vi "Comm@Write__Parameter.vi"(1 "ParamterIn":string) -> (0 "ParamterOut":string)   [LabVIEW 2019]
panel:
  in  "Message":string(combo)
  in  "Data2":string(combo) caption="Postfix"
  in  "Data1":string(combo) caption="Data"
  in  "CommName":string(combo)
  in  "Confirm":bool
  # "Comm@Write $Comm,$Data1,$Data2(,$[[label]]Message)"
  # "COM               $Data,$Postfix,$[[label]]Message)\nTCP                $Data,$Postfix,$[[label]]Message)\nServer              $Data,$Postfix,$[[label]]Message)\nModbus           $Address,$Data(,$[[label]]Message)\nModbus(TCP)   $Address,$Data(,$[[label]]Message)"
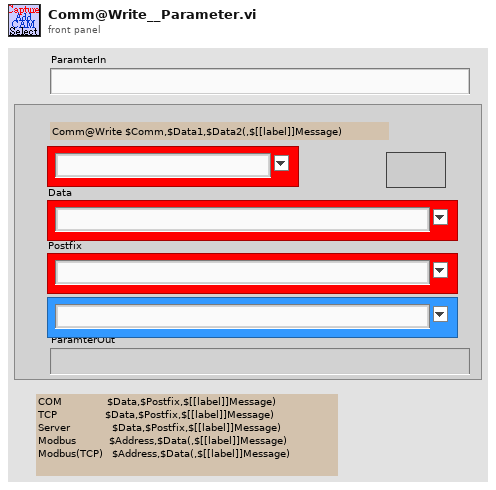
[diagram p1: front panel]
types:
  T1 = cluster{"Type":enum16{"COM", "TCP", "TCP(Slave)", "Modbus", "Modbus(TCP)", "COM(Slave)"}, "COMM":variant, "DataType":enum16{"ASCII", "Binary"}}
  T2 = enum16{"COM", "TCP", "TCP(Slave)", "Modbus", "Modbus(TCP)", "COM(Slave)"}
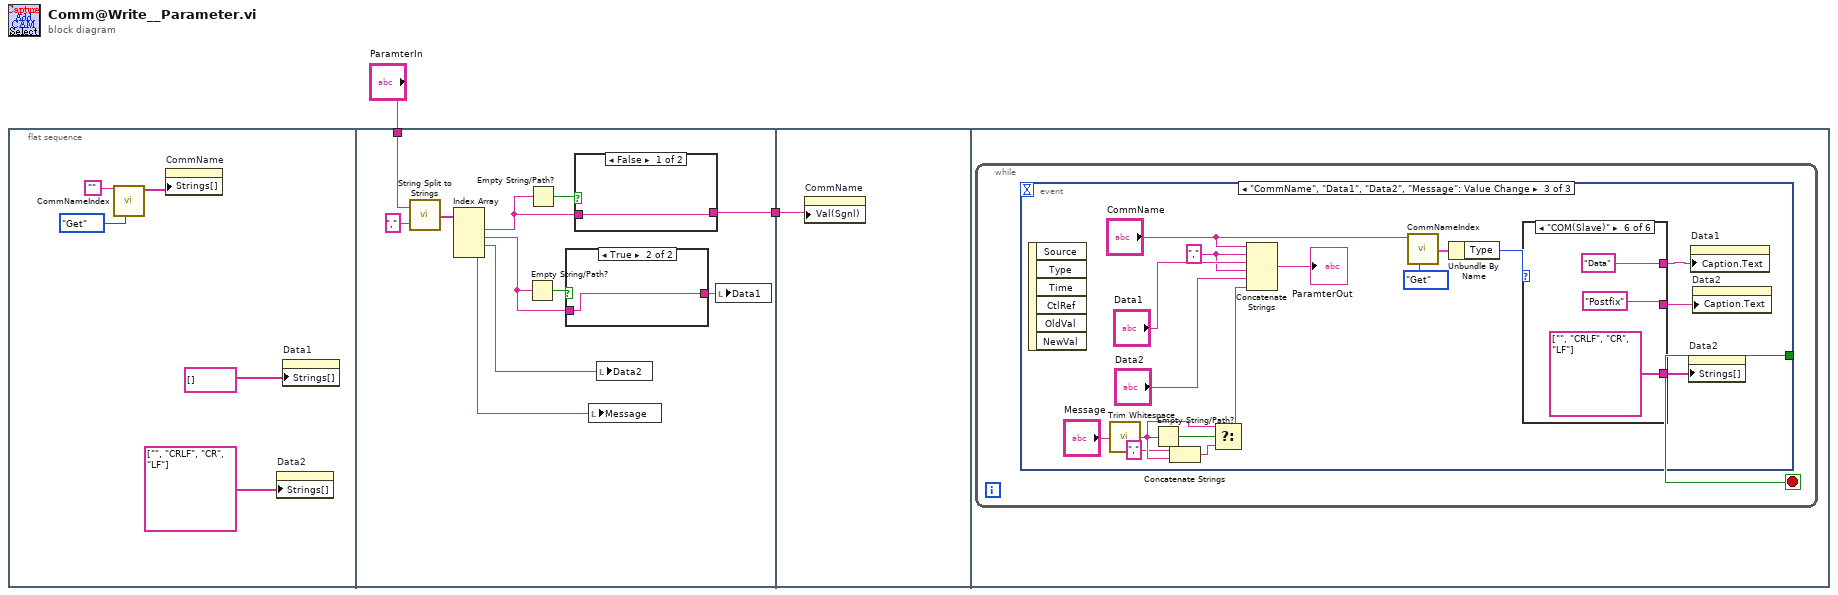
[diagram p0: block diagram]
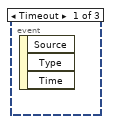
[diagram p4: hidden frame]
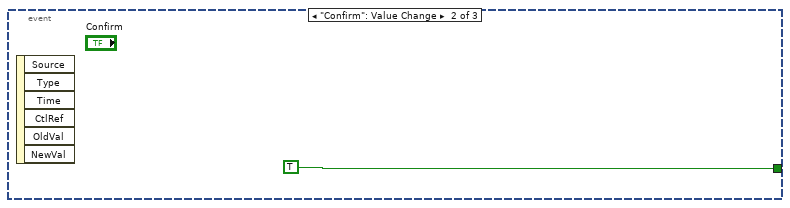
[diagram p5: hidden frame]
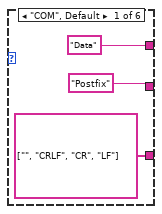
[diagram p6: hidden frame]
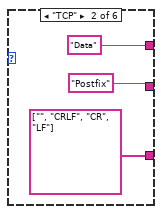
[diagram p7: hidden frame]
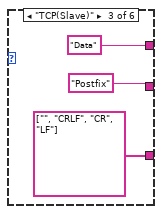
[diagram p8: hidden frame]
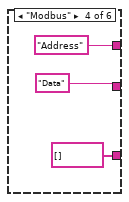
[diagram p9: hidden frame]
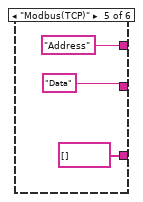
[diagram p10: hidden frame]
diagram:
  n1 = flat-sequence {
    tunnel: "ParamterIn" -> [w14]
    tunnel: [w16] -> w1
    tunnel: w1 -> [w23]
    frame #0 {
      n2 = call "CommNameIndex.vi"("OP"=enum16{"Init", "Get", "Set"}."Get", "Comm"="") -> ("CommNameS"=w5:string[])  [unwired: 7 in, 2 out]
      n3 = property on="CommName" class="CmbBox"("Strings[]"=w5) -> ()  [unwired: 2 in, 2 out]
      n4 = property on="Data2" class="CmbBox"("Strings[]"=string[] ["", "CRLF", "CR", "LF"] ("Strings []")) -> ()  [unwired: 2 in, 2 out]
      n5 = property on="Data1" class="CmbBox"("Strings[]"=string[] [] ("Strings []")) -> ()  [unwired: 2 in, 2 out]
    }
    frame #1 {
      n6 = call "String Split to Strings.vi"("search string/char (-)"=",", "String"=w14) -> ("Array"=w12:string[])
      n7 = Index Array(array=w12) -> (element #1=w11:string, element #2=w10:string, element #3=w9:string, element #4=w8:string)  [unwired: 4 in]
      n8 = Empty String/Path?(string/path=w10) -> (empty?=w17:bool)
      n9 = Empty String/Path?(string/path=w11) -> (empty?=w18:bool)
      n10 = case shown="True" w17 {
        tunnel: w10 -> [w19 w20]
        tunnel: [w19 w20] -> w15
        frame False {
        }
        frame True {
        }
      }
      n11 = case shown="False" w18 {
        tunnel: [w21 w22] -> w16
        tunnel: w11 -> [w21 w22]
        frame False {
        }
        frame True {
        }
      }
      n12 = local write "Message"(w8) -> ()
      n13 = local write "Data2"(w9) -> ()
      n14 = local write "Data1"(w15) -> ()
    }
    frame #2 {
      n15 = property on="CommName" class="CmbBox"("Val(Sgnl)"=w23) -> ()  [unwired: 2 in, 2 out]
    }
    frame #3 {
      n16 = while {
        stop <- w24 stop-if-true
        n17 = event shown="[2] \"CommName\", \"Data1\", \"Data2\", \"Message\": Value Change" {
          selector: _ -> [_ _ _]
          dyn-events: _ -> [_ _ _]
          timeout: _ -> [_ _ _]
          tunnel: [_ TRUE _] -> w24
          event Timeout {
            n18 = event-data() -> ()  [unwired: 1 in, 3 out]
          }
          event "Confirm": Value Change {
            n19 = event-data() -> ()  [unwired: 1 in, 6 out]
          }
          event "CommName", "Data1", "Data2", "Message": Value Change {
            w39 = "," ("string")
            n20 = event-data() -> ()  [unwired: 1 in, 6 out]
            n21 = call <vilib>:"Trim Whitespace.vi"("string"="Message") -> ("trimmed string"=w36:string)  [unwired: 1 in]
            n22 = Empty String/Path?(string/path=w36) -> (empty?=w37:bool)
            n23 = Concatenate Strings("," ("string"), w36) -> (w33:string)
            n24 = Select(t=w36, s=w37, f=w33) -> (s? t:f=w34:string)
            n25 = Concatenate Strings("CommName", w39, "Data1", w39, "Data2", w34) -> (→"ParamterOut":string)
            n26 = call "CommNameIndex.vi"("OP"=enum16{"Init", "Get", "Set"}."Get", "Comm"="CommName") -> ("DataOut"=w30:T1)  [unwired: 7 in, 2 out]
            n27 = Unbundle By Name(w30) -> ("Type"=w29:T2)
            n28 = case shown="\"COM(Slave)\"" w29 {
              tunnel: ["Data" "Data" "Data" "Address" "Address" "Data"] -> w28
              tunnel: ["Postfix" "Postfix" "Postfix" "Data" "Data" "Postfix"] -> w27
              tunnel: [string[] ["", "CRLF", "CR", "LF"] ("Strings []") string[] ["", "CRLF", "CR", "LF"] ("Strings []") string[] ["", "CRLF", "CR", "LF"] ("Strings []") string[] [] ("Strings []") string[] [] ("Strings []") string[] ["", "CRLF", "CR", "LF"] ("Strings []")] -> w26
              frame "COM", Default {
              }
              frame "TCP" {
              }
              frame "TCP(Slave)" {
              }
              frame "Modbus" {
              }
              frame "Modbus(TCP)" {
              }
              frame "COM(Slave)" {
              }
            }
            n29 = property on="Data2" class="CmbBox"("Strings[]"=w26) -> ()  [unwired: 2 in, 2 out]
            n30 = property on="Data1" class="CmbBox"("Caption.Text"=w28) -> ()  [unwired: 2 in, 2 out]
            n31 = property on="Data2" class="CmbBox"("Caption.Text"=w27) -> ()  [unwired: 2 in, 2 out]
          }
        }
      }
    }
  }
